vi "LEDs to Display.vi"(0 "Model Select":T1, 7 "Justice League UI":T9) -> (8 "JL Display":T2={"SSD"="", "Cycle Selection"=enum."Cycle 0", "Bar Selection"=enum."Bar 1", "Temp Setting"=enum."High", "Dryness Level"=enum."Extra Dry", "Time Setting"=enum."Default Time 5", "Dryer Status"=enum."Status 6", "Start/Pause"=FALSE, "Pause"=FALSE, "Control Lock"=FALSE, "Sensing"=FALSE, "Clean Filter"=FALSE, "My Cycle"=FALSE, "Delay Dry"=FALSE, "Volume"=FALSE, "Damp Alert"=FALSE, "Ext Tumble"=FALSE, "Decrement"=FALSE, "Increment"=FALSE, "eDry"=FALSE, "Extra Status"=FALSE})   [LabVIEW 2016]
uses:
  type defs/UI_LEDs.ctl
  type defs/JL Display.ctl
  type defs/Cycle Selection Enum.ctl
  type defs/Bar Enum.ctl
  type defs/Temp Setting Enum.ctl
  type defs/Dryness Enum.ctl
  type defs/Time Enum.ctl
  type defs/Status Enum.ctl
  type defs/JL_Trans-Model.ctl
  <vilib>/Utility/error.llb/whitespace.ctl
  type defs/JL_Trans-state.ctl
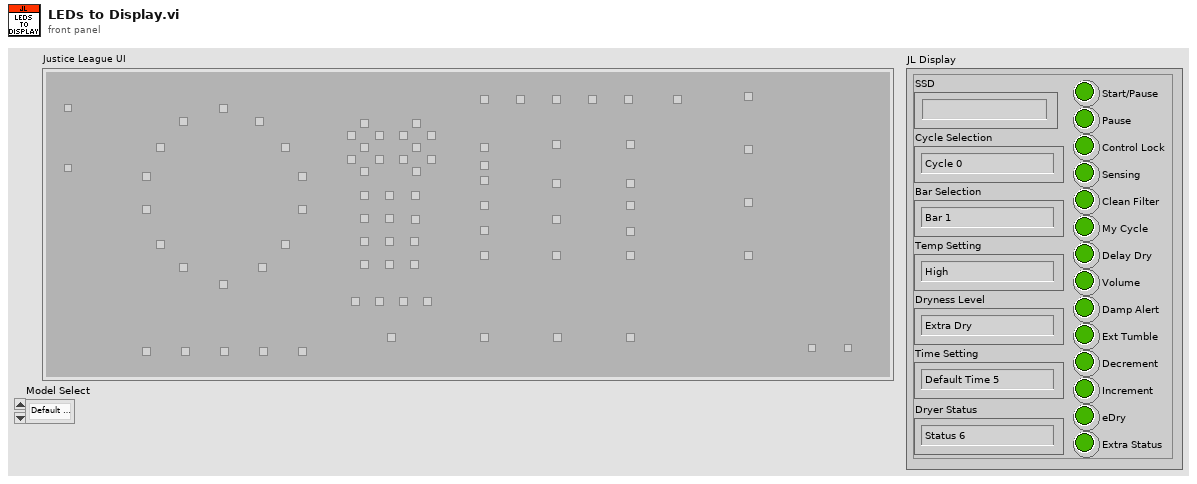
[diagram p1: front panel]
types:
  T1 = typedef "JL_Trans-Model.ctl" = enum16{"Default Model"}
  T2 = typedef "JL Display.ctl" = cluster{"SSD":string, "Cycle Selection":T3, "Bar Selection":T4, "Temp Setting":T5, "Dryness Level":T6, "Time Setting":T7, "Dryer Status":T8, "Start/Pause":bool, "Pause":bool, "Control Lock":bool, "Sensing":bool, "Clean Filter":bool, "My Cycle":bool, "Delay Dry":bool, "Volume":bool, "Damp Alert":bool, "Ext Tumble":bool, "Decrement":bool, "Increment":bool, "eDry":bool, "Extra Status":bool}
  T3 = typedef "Cycle Selection Enum.ctl" = enum16{"Cycle 0", "Cycle 1", "Cycle 2", "Cycle 3", "Cycle 4", "Cycle 5", "Cycle 6", "Cycle 7", "Cycle 8", "Cycle 9", "Cycle 10", "Cycle 11", "Cycle 12", "Cycle 13", "Off", "*Invalid"}
  T4 = typedef "Bar Enum.ctl" = enum16{"Bar 1", "Bar 2", "Bar 3", "Bar 4", "Bar 5", "Off", "*Incorrect*"}
  T5 = typedef "Temp Setting Enum.ctl" = enum16{"Off", "No Heat", "Extra Low", "Low", "Medium", "High", "*Incorrect*"}
  T6 = typedef "Dryness Enum.ctl" = enum16{"Off", "Damp", "Less Dry", "Dry", "More Dry", "Extra Dry", "*Incorrect*"}
  T7 = typedef "Time Enum.ctl" = enum16{"Off", "Default Time 1", "Default Time 2", "Default Time 3", "Default Time 4", "Default Time 5", "*Incorrect*"}
  T8 = typedef "Status Enum.ctl" = enum16{"Status 1", "Status 2", "Status 3", "Status 4", "Status 5", "Status 6", "Off", "*Incorrect*"}
  T9 = typedef "UI_LEDs.ctl" = cluster{"Z301 - Encoder 0":bool, "Z302 - Encoder 13":bool, "Z303 - Encoder 12":bool, "Z304 - Encoder 11":bool, "Z305 - Encoder 10":bool, "Z306 - Encoder 09":bool, "Z307 - Encoder 08":bool, "Z308 - Encoder 07":bool, "Z309 - Encoder 06":bool, "Z310 - Encoder 05":bool, "Z311 - Encoder 04":bool, "Z312 - Encoder 03":bool, "Z313 - Encoder 02":bool, "Z314 - Encoder 01":bool, "Z315 - Unpopulated":bool, "Z316 - Unpopulated":bool, "Z317 - SSD1:A":bool, "Z318 - SSD1:B":bool, "Z319 - SSD1:G":bool, "Z320 - SSD1:C":bool, "Z321 - SSD1:D":bool, "Z322 - SSD1:E":bool, "Z323 - SSD1:F":bool, "Z324 - Pause 1":bool, "Z325 - Control Lock 1":bool, "Z326 - Sensing 1":bool, "Z327 - Clean Lint Filter 1":bool, "Z328 - Extra Status 1":bool, "Z329 - Extra Status 2":bool, "Z330 - Clean Lint Filter 2":bool, "Z331 -Sensing 2":bool, "Z332 - Unpopulated":bool, "Z333 - SSD2:A":bool, "Z334 - SSD2:B":bool, "Z335 - SSD2:G":bool, "Z345 - SSD2:C":bool, "Z336 - SSD2:D":bool, "Z337 - SSD2:E":bool, "Z338 - SSD2:F":bool, "Z339 - Pause 3":bool, "Z340 - Control Lock 3":bool, "Z353 - Sensing 3":bool, "Z342 - Clean Lint Filter 3":bool, "Z344 - Extra Status 3":bool, "Z346 - Extra Status 4":bool, "Z341 - Pause 2":bool, "Z343 - Control Lock 2":bool, "Z347 - Unpopulated":bool, "Z348 -My Cycle":bool, "Z349 - Delay Dry":bool, "Z350 - Volume":bool, "Z351 - Damp Alert":bool, "Z352 - Bar 1":bool, "Z354 - Bar 2":bool, "Z355 - Bar 3":bool, "Z356 - Bar 4":bool, "Z357 - Bar 5":bool, "Z358 - eDry":bool, "Z359 - Time Increment":bool, "Z360 - Time Decrement":bool, "Z361 - Extended Tumble":bool, "Z362 - Unpopulated":bool, "Z363 - Unpopulated":bool, "Z364 - Unpopulated":bool, "Z365 - Status 1":bool, "Z366 - Status 3":bool, "Z367 - Default Time 5":bool, "Z368 - Default Time 4":bool, "Z369 - Default Time 3":bool, "Z370 - Dry":bool, "Z371 - Status 2":bool, "Z372 -Default Time 2":bool, "Z373 - Default Time 1":bool, "Z374 - Unpopulated":bool, "Z375 - Default Time 0":bool, "Z376 - No Heat":bool, "Z377 - Unpopulated":bool, "Z378 - Unpopulated":bool, "Z379 - Unpopulated":bool, "Z380 - Unpopulated":bool, "Z381 - Status 4":bool, "Z382 - Status 6":bool, "Z383 - More Dry":bool, "Z384 - High":bool, "Z385 - Medium":bool, "Z386 -Low":bool, "Z387 - Status 5":bool, "Z388 - Less Dry":bool, "Z388 - Extra Low":bool, "Z390 - Unpopulated":bool, "Z391 - Damp":bool, "Z392 - Unpopulated":bool, "Z393 - Unpopulated":bool, "Z394 - Unpopulated":bool, "Z395 - Unpopulated":bool, "Z396 - Unpopulated":bool, "Z101 - unpop?":bool, "Z102 - Start/Pause":bool, "OFF - OFF":bool, "MAX - MAX":bool}
  T10 = typedef "JL_Trans-state.ctl" = enum16{"Temp ", "Time", "Level", "stop"}
  T11 = typedef "whitespace.ctl" = u16
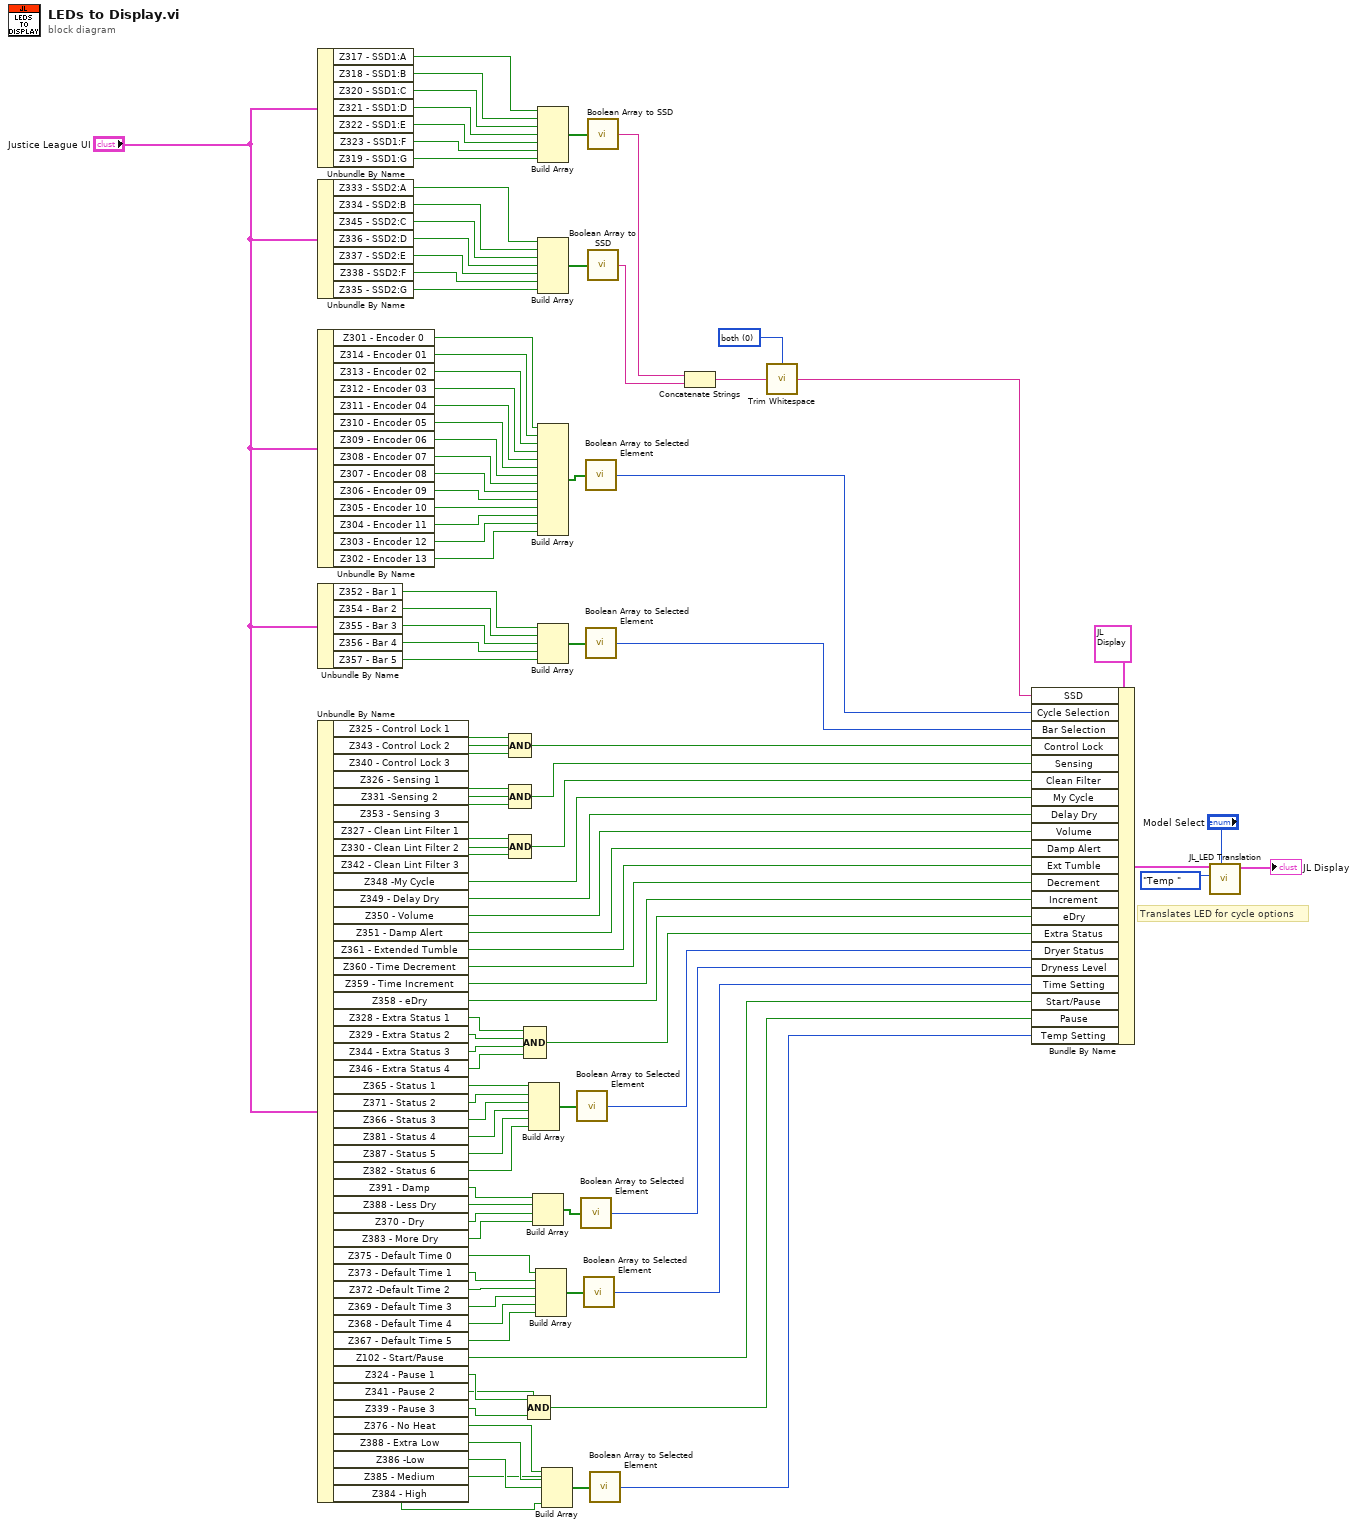
[diagram p0: block diagram]
diagram:
  w5 = T11 0 items=["both", "start of string", "end of string"] ("location (both)")
  # "Translates LED for cycle options"
  n1 = Unbundle By Name("Justice League UI") -> ("Z317 - SSD1:A"=w61:bool, "Z318 - SSD1:B"=w62:bool, "Z320 - SSD1:C"=w63:bool, "Z321 - SSD1:D"=w64:bool, "Z322 - SSD1:E"=w65:bool, "Z323 - SSD1:F"=w66:bool, "Z319 - SSD1:G"=w67:bool)
  n2 = Unbundle By Name("Justice League UI") -> ("Z333 - SSD2:A"=w109:bool, "Z334 - SSD2:B"=w108:bool, "Z345 - SSD2:C"=w107:bool, "Z336 - SSD2:D"=w106:bool, "Z337 - SSD2:E"=w105:bool, "Z338 - SSD2:F"=w104:bool, "Z335 - SSD2:G"=w103:bool)
  n3 = Unbundle By Name("Justice League UI") -> ("Z301 - Encoder 0"=w100:bool, "Z314 - Encoder 01"=w99:bool, "Z313 - Encoder 02"=w98:bool, "Z312 - Encoder 03"=w97:bool, "Z311 - Encoder 04"=w96:bool, "Z310 - Encoder 05"=w95:bool, "Z309 - Encoder 06"=w94:bool, "Z308 - Encoder 07"=w93:bool, "Z307 - Encoder 08"=w92:bool, "Z306 - Encoder 09"=w91:bool, "Z305 - Encoder 10"=w90:bool, "Z304 - Encoder 11"=w89:bool, "Z303 - Encoder 12"=w88:bool, "Z302 - Encoder 13"=w58:bool)
  n4 = Unbundle By Name("Justice League UI") -> ("Z352 - Bar 1"=w87:bool, "Z354 - Bar 2"=w86:bool, "Z355 - Bar 3"=w85:bool, "Z356 - Bar 4"=w84:bool, "Z357 - Bar 5"=w83:bool)
  n5 = Unbundle By Name("Justice League UI") -> ("Z325 - Control Lock 1"=w80:bool, "Z343 - Control Lock 2"=w79:bool, "Z340 - Control Lock 3"=w78:bool, "Z326 - Sensing 1"=w77:bool, "Z331 -Sensing 2"=w76:bool, "Z353 - Sensing 3"=w75:bool, "Z327 - Clean Lint Filter 1"=w74:bool, "Z330 - Clean Lint Filter 2"=w73:bool, "Z342 - Clean Lint Filter 3"=w72:bool, "Z348 -My Cycle"=w53:bool, "Z349 - Delay Dry"=w52:bool, "Z350 - Volume"=w51:bool, "Z351 - Damp Alert"=w50:bool, "Z361 - Extended Tumble"=w49:bool, "Z360 - Time Decrement"=w48:bool, "Z359 - Time Increment"=w47:bool, "Z358 - eDry"=w46:bool, "Z328 - Extra Status 1"=w44:bool, "Z329 - Extra Status 2"=w43:bool, "Z344 - Extra Status 3"=w42:bool, "Z346 - Extra Status 4"=w45:bool, "Z365 - Status 1"=w39:bool, "Z371 - Status 2"=w38:bool, "Z366 - Status 3"=w37:bool, "Z381 - Status 4"=w36:bool, "Z387 - Status 5"=w35:bool, "Z382 - Status 6"=w34:bool, "Z391 - Damp"=w31:bool, "Z388 - Less Dry"=w30:bool, "Z370 - Dry"=w29:bool, "Z383 - More Dry"=w28:bool, "Z375 - Default Time 0"=w25:bool, "Z373 - Default Time 1"=w24:bool, "Z372 -Default Time 2"=w23:bool, "Z369 - Default Time 3"=w22:bool, "Z368 - Default Time 4"=w21:bool, "Z367 - Default Time 5"=w20:bool, "Z102 - Start/Pause"=w18:bool, "Z324 - Pause 1"=w17:bool, "Z341 - Pause 2"=w16:bool, "Z339 - Pause 3"=w15:bool, "Z376 - No Heat"=w11:bool, "Z388 - Extra Low"=w10:bool, "Z386 -Low"=w9:bool, "Z385 - Medium"=w8:bool, "Z384 - High"=w7:bool)
  n6 = Compound Arithmetic op=AND(w80, w79, w78) -> (w57:bool)
  n7 = Compound Arithmetic op=AND(w77, w76, w75) -> (w55:bool)
  n8 = Compound Arithmetic op=AND(w74, w73, w72) -> (w54:bool)
  n9 = Compound Arithmetic op=AND(w44, w43, w42, w45) -> (w41:bool)
  n10 = Compound Arithmetic op=AND(w17, w16, w15) -> (w14:bool)
  n11 = Build Array(w39, w38, w37, w36, w35, w34) -> (w40:bool[])
  n12 = Build Array(w31, w30, w29, w28) -> (w32:bool[])
  n13 = Build Array(w25, w24, w23, w22, w21, w20) -> (w26:bool[])
  n14 = Build Array(w61, w62, w63, w64, w65, w66, w67) -> (w68:bool[])
  n15 = Build Array(w109, w108, w107, w106, w105, w104, w103) -> (w102:bool[])
  n16 = Build Array(w100, w99, w98, w97, w96, w95, w94, w93, w92, w91, w90, w89, w88, w58) -> (w81:bool[])
  n17 = Build Array(w87, w86, w85, w84, w83) -> (w82:bool[])
  n18 = Build Array(w11, w10, w9, w8, w7) -> (w13:bool[])
  n19 = call "Boolean Array to Selected Element.vi"("Bool Array In"=w40) -> ("Selected Element Out"=w33:i32)  [unwired: 14 in]
  n20 = call "Boolean Array to Selected Element.vi"("Bool Array In"=w32) -> ("Selected Element Out"=w27:i32)  [unwired: 14 in]
  n21 = call "Boolean Array to Selected Element.vi"("Bool Array In"=w26) -> ("Selected Element Out"=w19:i32)  [unwired: 14 in]
  n22 = call "Boolean Array to Selected Element.vi"("Bool Array In"=w81) -> ("Selected Element Out"=w70:i32)  [unwired: 14 in]
  n23 = call "Boolean Array to Selected Element.vi"("Bool Array In"=w82) -> ("Selected Element Out"=w71:i32)  [unwired: 14 in]
  n24 = call "Boolean Array to SSD.vi"("7 Segment Bool Array In"=w68) -> ("7 Segment Out"=w60:string)  [unwired: 14 in]
  n25 = call "Boolean Array to SSD.vi"("7 Segment Bool Array In"=w102) -> ("7 Segment Out"=w101:string)  [unwired: 14 in]
  n26 = call "Boolean Array to Selected Element.vi"("Bool Array In"=w13) -> ("Selected Element Out"=w12:i32)  [unwired: 14 in]
  n27 = Concatenate Strings(w60, w101) -> (w69:string)
  n28 = call <vilib>:"Trim Whitespace.vi"("string"=w69, "location (both)"=w5) -> ("trimmed string"=w6:string)
  n29 = Bundle By Name(cluster=T2 {"SSD"="", "Cycle Selection"=enum."Cycle 0", "Bar Selection"=enum."Bar 1", "Temp Setting"=enum."High", "Dryness Level"=enum."Extra Dry", "Time Setting"=enum."Default Time 5", "Dryer Status"=enum."Status 6", "Start/Pause"=FALSE, "Pause"=FALSE, "Control Lock"=FALSE, "Sensing"=FALSE, "Clean Filter"=FALSE, "My Cycle"=FALSE, "Delay Dry"=FALSE, "Volume"=FALSE, "Damp Alert"=FALSE, "Ext Tumble"=FALSE, "Decrement"=FALSE, "Increment"=FALSE, "eDry"=FALSE, "Extra Status"=FALSE} ("JL Display"), "SSD"=w6, "Cycle Selection"=w70, "Bar Selection"=w71, "Control Lock"=w57, "Sensing"=w55, "Clean Filter"=w54, "My Cycle"=w53, "Delay Dry"=w52, "Volume"=w51, "Damp Alert"=w50, "Ext Tumble"=w49, "Decrement"=w48, "Increment"=w47, "eDry"=w46, "Extra Status"=w41, "Dryer Status"=w33, "Dryness Level"=w27, "Time Setting"=w19, "Start/Pause"=w18, "Pause"=w14, "Temp Setting"=w12) -> (w4:T2)
  n30 = call "JL_LED Translation.vi"("Model Select"="Model Select", "Option"=JL_Trans-state."Temp ", "JL Display"=w4) -> ("JL Display 2"=→"JL Display":T2)  [unwired: 7 in, 1 out]
